vi "SVL Decimated Exp Avg Sound Level.vi"   [LabVIEW 2017, in "SoundVib_SoundLevel.lvlib"]
doc: "Computes the exponential averaged sound level of <B>scaled signal [EU]</B> based on <B>exponential mode</B>, decimates this sound level by <B>decimation factor</B>, and returns the result in <B>decimated exp avg sound level [dB EU]</B>. You can use this polymorphic VI to compute the exponential averaged sound level for a single channel or for N channels. The data type you wire to the <B>scaled signal [EU]</B> input determines the polymorphic instance to use."
uses:
  <vilib>/addons/Sound and Vibration/svt_Level/SoundVib_SoundLevel.lvlib
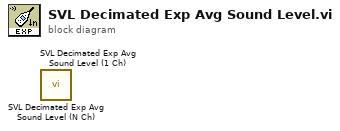
[diagram p0: block diagram]
diagram:
  n1 = call <vilib>:"SVL Decimated Exp Avg Sound Level (N Ch).vi"() -> ()  [unwired: 7 in, 5 out]
  n2 = call <vilib>:"SVL Decimated Exp Avg Sound Level (1 Ch).vi"() -> ()  [unwired: 7 in, 5 out]
